vi "2020_day01.vi"() -> ()   [LabVIEW 2021]
panel:
  out "Result 2":i32
  out "Result":i32
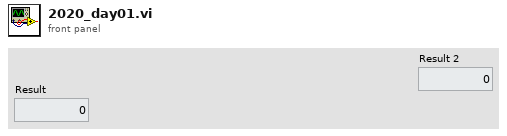
[diagram p1: front panel]
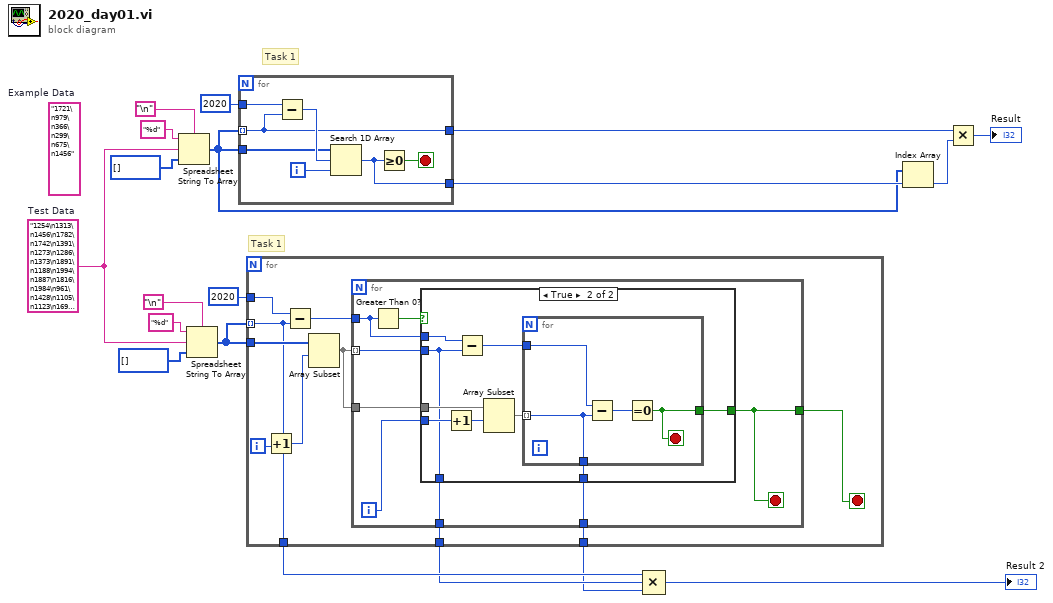
[diagram p0: block diagram]
diagram:
  w1 = "1254\n1313\n1456\n1782\n1742\n1391\n1273\n1286\n1373\n1891\n1188\n1994\n1887\n1816\n1984\n961\n1428\n1105\n1123\n1699\n1154\n1953\n1977\n1450\n1696\n1068\n1241\n1926\n1228\n1591\n1789\n1966\n1508\n1193\n1190\n1654\n444\n1282\n1169\n1165\n1778\n1669\n1570\n1671\n1845\n1208\n1728\n1798\n847\n1300\n1817\n1200\n1297\n1658\n1296\n1571\n1991\n1305\n1314\n1903\n1472\n1359\n1506\n1999\n1877\n1168\n1137\n1288\n1083\n1656\n413\n1430\n1408\n1397\n1846\n1218\n684\n1234\n2007\n900\n1604\n1460\n1848\n1693\n1324\n1401\n1968\n1918\n1975\n1665\n1413\n1874\n1852\n1521\n1753\n1229\n1940\n1650\n1976\n1235\n1130\n1927\n1365\n1908\n1441\n1302\n1986\n1449\n1692\n1944\n1277\n1312\n1826\n1231\n1289\n1814\n1170\n1606\n1608\n1773\n1883\n1936\n1626\n1497\n1860\n1673\n1295\n2005\n1481\n1995\n1734\n1646\n1557\n1298\n1174\n1894\n1309\n1240\n1982\n1414\n1799\n1620\n1863\n1220\n1642\n508\n1146\n1187\n1253\n1284\n1952\n1527\n1610\n1333\n1221\n1362\n1457\n1721\n1493\n1330\n156\n1647\n1841\n1724\n2000\n1398\n1745\n1985\n1269\n1722\n2001\n1923\n1395\n1094\n1140\n1958\n1239\n1336\n1588\n1338\n1750\n1757\n1444\n1822\n1335\n1941\n1865\n1767\n1881\n1499\n1157\n1990\n1210\n1779\n1201\n1784\n1961\n1476\n1861"  # Test Data
  (unwired) "1721\n979\n366\n299\n675\n1456"  # Example Data
  # "Task 1"
  # "Task 1"
  n1 = Spreadsheet String To Array(delimiter (Tab)="\n", format string="%d", spreadsheet string=w1, array type (2D Dbl)=i32[] []) -> (array=w12:i32[])
  n2 = Spreadsheet String To Array(delimiter (Tab)="\n", format string="%d", spreadsheet string=w1, array type (2D Dbl)=i32[] []) -> (array=w10:i32[])
  n3 = for {
    tunnel: w12 -> [w24]
    tunnel: w12 -> [w22] mode=indexing
    tunnel: 2020 -> [w26]
    tunnel: [w22] -> w15
    tunnel: [w20] -> w14
    i -> [w21]
    stop <- w23 stop-if-true
    n4 = Subtract(x=w26, y=w22) -> (x-y=w25:i32)
    n5 = Search 1D Array(1D array=w24, element=w25, start index (0)=w21) -> (index of element=w20:i32)
    n6 = Greater Or Equal To 0?(x=w20) -> (x >= 0?=w23:bool)
  }
  n7 = for {
    tunnel: w10 -> [w34]
    tunnel: w10 -> [w29] mode=indexing
    tunnel: 2020 -> [w36]
    tunnel: [w29] -> w5
    tunnel: [w28] -> w4
    tunnel: [w27] -> w3
    i -> [w33]
    stop <- w30 stop-if-true
    n8 = Increment(x=w33) -> (x+1=w32:i32)
    n9 = Subtract(x=w36, y=w29) -> (x-y=w35:i32)
    n10 = Array Subset(array=w34, index=w32) -> (w31:i32[])  [unwired: 1 in]
    n11 = for {
      tunnel: w35 -> [w42]
      tunnel: w31 -> [w43] mode=indexing
      tunnel: w31 -> [w40]
      tunnel: [w39] -> w30
      tunnel: [w38] -> w28
      tunnel: [w37] -> w27
      i -> [w41]
      stop <- w39 stop-if-true
      n12 = Greater Than 0?(x=w42) -> (x > 0?=w44:bool)
      n13 = case shown="True" w44 {
        tunnel: w43 -> [_ w46]
        tunnel: w42 -> [_ w53]
        tunnel: w41 -> [_ w52]
        tunnel: w40 -> [_ w49]
        tunnel: [_ w47] -> w39
        tunnel: [_ w46] -> w38
        tunnel: [_ w45] -> w37
        frame False {
        }
        frame True {
          n14 = Increment(x=w52) -> (x+1=w51:i32)
          n15 = Subtract(x=w53, y=w46) -> (x-y=w48:i32)
          n16 = Array Subset(array=w49, index=w51) -> (w50:i32[])  [unwired: 1 in]
          n17 = for {
            tunnel: w50 -> [w54] mode=indexing
            tunnel: w48 -> [w57]
            tunnel: [w55] -> w47
            tunnel: [w54] -> w45
            stop <- w55 stop-if-true
            n18 = Subtract(x=w57, y=w54) -> (x-y=w56:i32)
            n19 = Equal To 0?(x=w56) -> (x = 0?=w55:bool)
          }
        }
      }
    }
  }
  n20 = Compound Arithmetic op=MULTIPLY(w5, w4, w3) -> (→"Result 2":i32)
  n21 = Index Array(array=w12, index=w14) -> (element=w13:i32)
  n22 = Multiply(x=w15, y=w13) -> (x*y=→"Result":i32)
